vi "Format Headers.vi"(1 "Headers":variant) -> (0 "Headers":string)   [LabVIEW 2023, in "Response.lvclass"]
uses:
  Response.lvclass
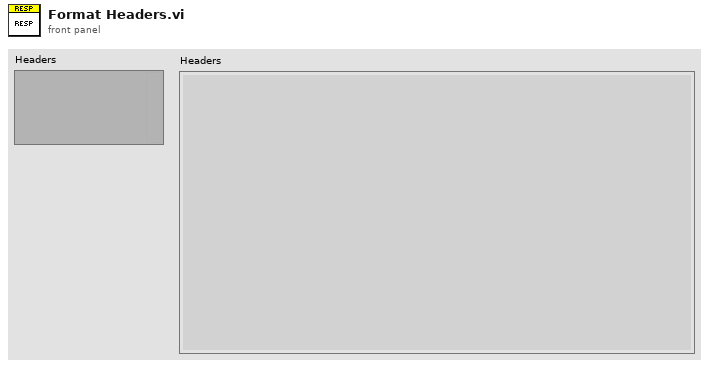
[diagram p1: front panel]
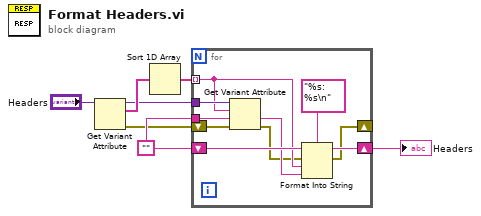
[diagram p0: block diagram]
diagram:
  w3 = ""
  n1 = Get Variant Attribute(Variant="Headers") -> (duplicate Variant=w4:variant, names=w6:string[], error out=w2:errorcluster)  [unwired: 3 in, 1 out]
  n2 = Sort 1D Array(array=w6) -> (sorted array=w5:string[])
  n3 = for {
    tunnel: w5 -> [w14] mode=indexing
    tunnel: w4 -> [w17]
    shift-right: [w15] -> w1
    shift-left: w3 -> [w16]
    tunnel: w3 -> [w12]
    shift-right: [w9] -> _
    shift-left: w2 -> [w10]
    n4 = Get Variant Attribute(Variant=w17, name=w14, default value (empty Variant)=w12, error in=w10) -> (value=w13:string, error out=w11:errorcluster)  [unwired: 2 out]
    n5 = Format Into String(format string="%s: %s\n", initial string=w16, error in=w11, w14, w13) -> (resulting string=w15:string, error out=w9:errorcluster)
  }
  "Headers" <- w1
